vi "ReadSelectivePacket.vi"(2 "Filename":string, 3 "NXT":T2={"Hardware"="NXT", "Flattened String"=""}) -> (0 "NXT":T2={"Hardware"="NXT", "Flattened String"=""}, 1 "Button Data":string, 5 "Joystick Data":string, 6 "Aux. Data":string, 7 "Time (MS)":u32, 9 "Packet Type":T1(ring), 10 "EOF":bool)   [LabVIEW 2010, in "Packet Recorder.lvlib"]
uses:
  Packet Recorder.lvlib
  <vilib>/NXT/Subs/LVHSConnector.ctl
  <vilib>/NXT/Dual Mode Library/prims/sign/sign_int.vi
panel:
  out "#Joystick Bytes":u8
  out "#Button Bytes":u8
  in  "Stored Filename":string
  in  "Stored Time":i32
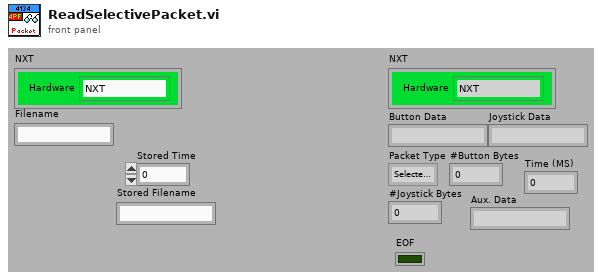
[diagram p1: front panel]
types:
  T1 = enum16{"Selected Joysticks", "Selected Buttons", "Selected Buttons and Joysticks", "Custom Call (w/ Aux. Data)"}
  T2 = typedef "LVHSConnector.ctl" = cluster{"Hardware":string, "Flattened String":string}
  T3 = enum16{"big-endian, network order", "native, host order", "little-endian"}
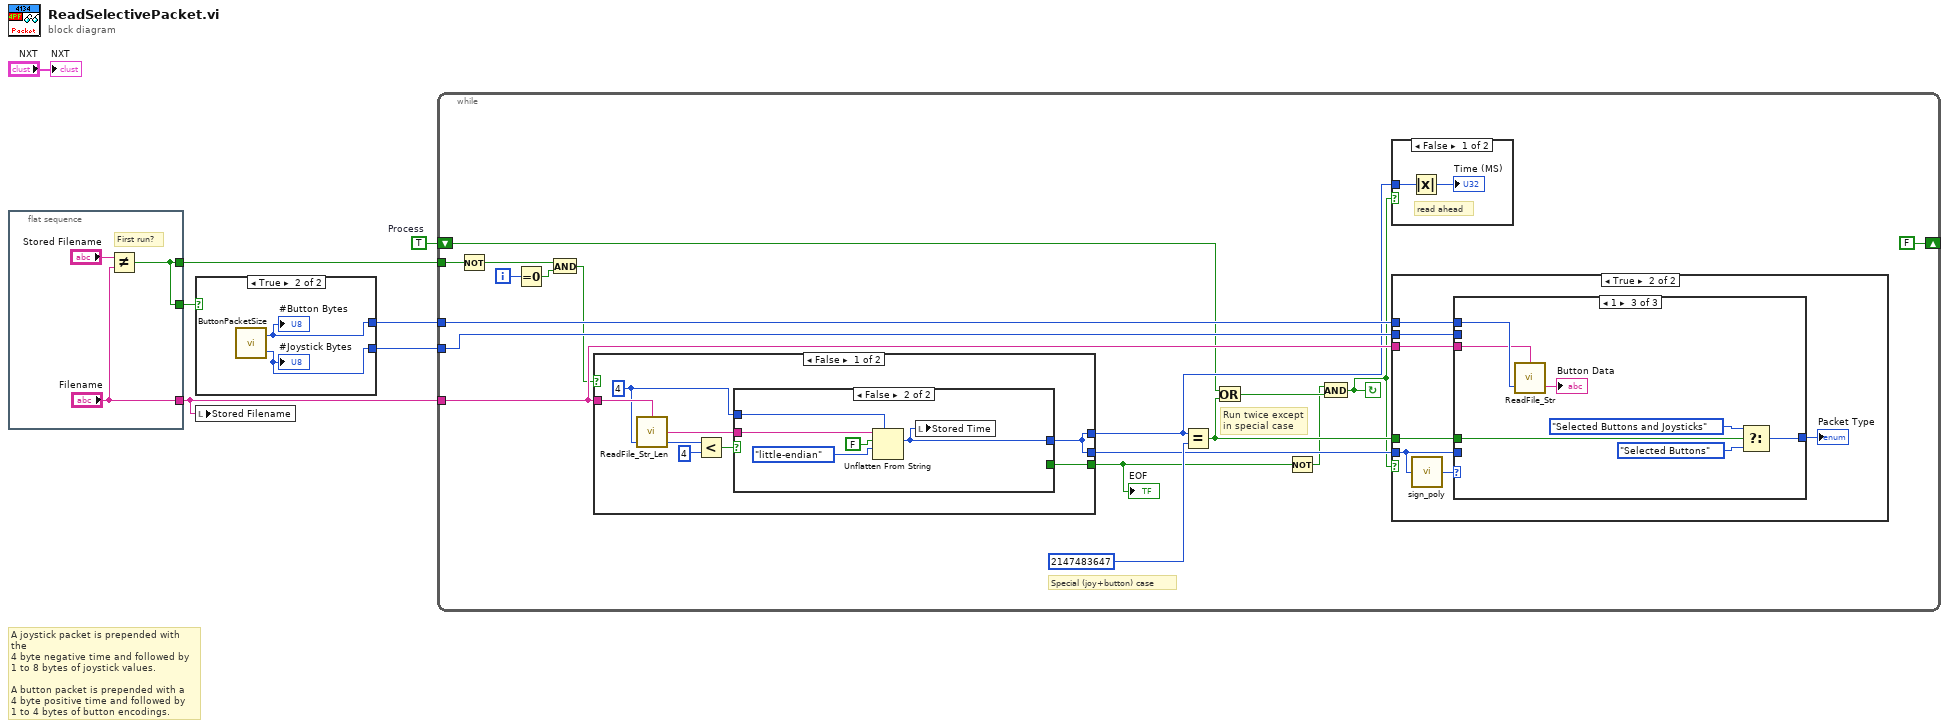
[diagram p0: block diagram]
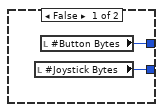
[diagram p2: hidden frame]
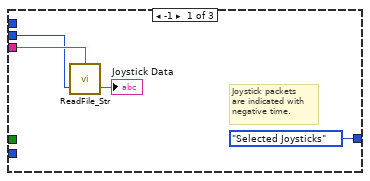
[diagram p5: hidden frame]
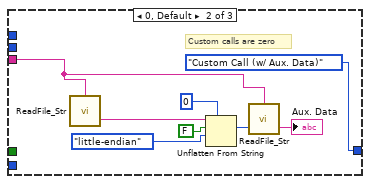
[diagram p6: hidden frame]
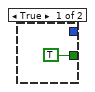
[diagram p7: hidden frame]
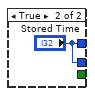
[diagram p8: hidden frame]
diagram:
  w4 = TRUE  # Process
  # "A joystick packet is prepended with the\n4 byte negative time and followed by\n1 to 8 bytes of joystick values.\n\nA button packet is prepended with a\n4 byte positive time and followed by\n1 to 4 bytes of button encodings."
  n1 = flat-sequence {
    tunnel: ["Filename"] -> w6
    tunnel: [w8] -> w5
    tunnel: [w8] -> w3
    frame #0 {
      # "First run?"
      n2 = Not Equal?(x="Stored Filename", y="Filename") -> (x != y?=w8:bool)
    }
  }
  n3 = case shown="True" w3 {
    tunnel: [w12 w13] -> w2
    tunnel: [w11 w14] -> w1
    frame False {
      n4 = local read "#Joystick Bytes"() -> (w11:u8)
      n5 = local read "#Button Bytes"() -> (w12:u8)
    }
    frame True {
      n6 = call "ButtonPacketSize.vi"() -> ("joystick packet size"=w14:u8, "button packet size"=w13:u8)  [unwired: 2 in]
      "#Button Bytes" <- w13
      "#Joystick Bytes" <- w14
    }
  }
  n7 = local write "Stored Filename"(w6) -> ()
  n8 = while {
    tunnel: w6 -> [w26]
    tunnel: w5 -> [w24]
    shift-right: [FALSE ("Process")] -> _
    shift-left: w4 -> [w19]
    tunnel: w2 -> [w28]
    tunnel: w1 -> [w27]
    i -> [w16]
    stop <- w15 continue-if-true
    # "Special (joy+button) case"
    # "Run twice except\nin special case"
    n9 = Not(x=w24) -> (.not. x?=w23:bool)
    n10 = Equal To 0?(x=w16) -> (x = 0?=w22:bool)
    n11 = And(x=w23, y=w22) -> (x .and. y?=w25:bool)
    n12 = case shown="False" w25 {
      tunnel: [w68 "Stored Time"] -> w29
      tunnel: w26 -> [w64 _]
      tunnel: [w68 "Stored Time"] -> w21
      tunnel: [w67 _] -> w20
      frame False {
        w63 = 4 ("Length (1)")
        n13 = call "ReadFile_Str_Len.vi"("Length (1)"=w63, "Filename"=w64) -> ("Length"=w61:u32, "String"=w62:string)  [unwired: 1 in, 1 out]
        n14 = Less?(x=w61, y=4) -> (x < y?=w66:bool)
        n15 = case shown="False" w66 {
          tunnel: w63 -> [_ w74]
          tunnel: [_ w71] -> w68
          tunnel: w62 -> [_ w70]
          tunnel: [TRUE ("EOF") _] -> w67
          frame True {
          }
          frame False {
            n16 = Unflatten From String(type=w74, binary string=w70, data includes array or string size? (T)=FALSE, byte order (0:big-endian, network order)=T3."little-endian") -> (value=w71:i32)  [unwired: 1 in, 2 out]
            n17 = local write "Stored Time"(w71) -> ()
          }
        }
      }
      frame True {
      }
    }
    "EOF" <- w20
    n18 = Equal?(x=w21, y=2147483647) -> (x = y?=w30:bool)
    n19 = Or(x=w19, y=w30) -> (x .or. y?=w18:bool)
    n20 = Not(x=w20) -> (.not. x?=w17:bool)
    n21 = And(x=w17, y=w18) -> (x .and. y?=w15:bool)
    n22 = case shown="False" w15 {
      tunnel: w21 -> [w33 _]
      frame False {
        # "read ahead"
        n23 = Absolute Value(x=w33) -> (abs(x)=→"Time (MS)":i32)
      }
      frame True {
      }
    }
    n24 = case shown="True" w15 {
      tunnel: w29 -> [_ w41]
      tunnel: w30 -> [_ w39]
      tunnel: w28 -> [_ w38]
      tunnel: w27 -> [_ w37]
      tunnel: w26 -> [_ w36]
      frame False {
      }
      frame True {
        n25 = call-poly <vilib>:"sign_poly.vi"("number"=w41) -> ("-1, 0, 1"=w40:i32)  [unwired: 4 in]
        n26 = case shown="1" w40 {
          tunnel: [T1."Selected Joysticks" ("Packet Type") T1."Custom Call (w/ Aux. Data)" ("Packet Type") w57] -> w35
          tunnel: w41 -> [_ _ _]
          tunnel: w39 -> [_ _ w60]
          tunnel: w38 -> [_ _ w56]
          tunnel: w37 -> [w43 _ _]
          tunnel: w36 -> [w44 w47 w55]
          frame -1 {
            # "Joystick packets\nare indicated with\nnegative time."
            n27 = call <vilib>:"ReadFile_Str.vi"("Length (1)"=w43, "Filename"=w44) -> ("String"=→"Joystick Data":string)  [unwired: 1 in, 1 out]
          }
          frame 0, Default {
            # "Custom calls are zero"
            n28 = call <vilib>:"ReadFile_Str.vi"("Filename"=w47) -> ("String"=w51:string)  [unwired: 2 in, 1 out]
            n29 = Unflatten From String(type=u8 0, binary string=w51, data includes array or string size? (T)=FALSE, byte order (0:big-endian, network order)=T3."little-endian") -> (value=w48:u8)  [unwired: 1 in, 2 out]
            n30 = call <vilib>:"ReadFile_Str.vi"("Length (1)"=w48, "Filename"=w47) -> ("String"=→"Aux. Data":string)  [unwired: 1 in, 1 out]
          }
          frame 1 {
            n31 = call <vilib>:"ReadFile_Str.vi"("Length (1)"=w56, "Filename"=w55) -> ("String"=→"Button Data":string)  [unwired: 1 in, 1 out]
            n32 = Select(t=T1."Selected Buttons and Joysticks" ("Packet Type"), s=w60, f=T1."Selected Buttons" ("Packet Type")) -> (s? t:f=w57:T1)
          }
        }
        "Packet Type" <- w35
      }
    }
  }
  "NXT" <- "NXT"
